vi "飞行姿态模拟.vi"() -> ()   [LabVIEW 2014]
uses:
  <vilib>/Utility/miscctls.llb/LVRGBAColorTypeDef.ctl
  <vilib>/picture/3D Picture Control/Object/Create Object (name).vi
  <vilib>/picture/3D Picture Control/Object/Add Object (reference).vi
  <vilib>/picture/3D Picture Control/NI_3D Picture Control.lvlib
panel:
  in  "退出按钮":bool
  in  "Yaw":dbl(knob) scale=-180.0..180.0
  in  "Roll":dbl(knob) scale=-90.0..90.0
  in  "Pitch":dbl(knob) scale=-180.0..180.0
  out "三维图片":refnum<vi>(3d-picture)
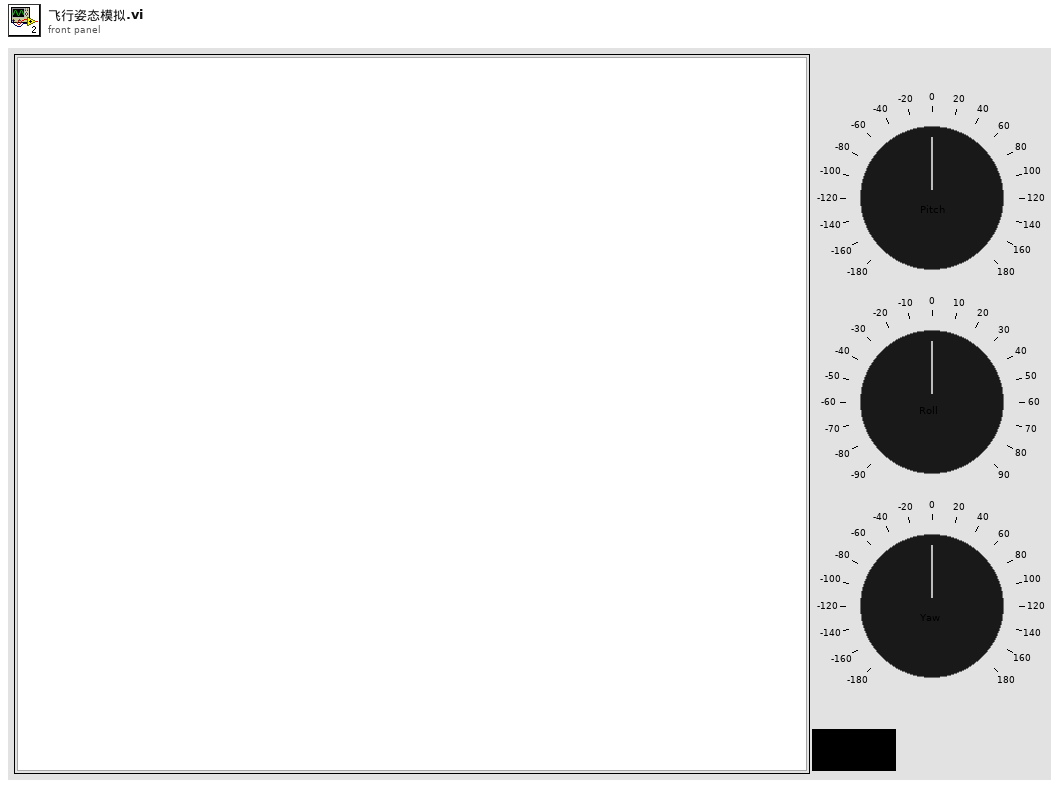
[diagram p1: front panel]
types:
  T1 = typedef "LVRGBAColorTypeDef.ctl" = cluster{"Red":sgl, "Green":sgl, "Blue":sgl, "Alpha":sgl}
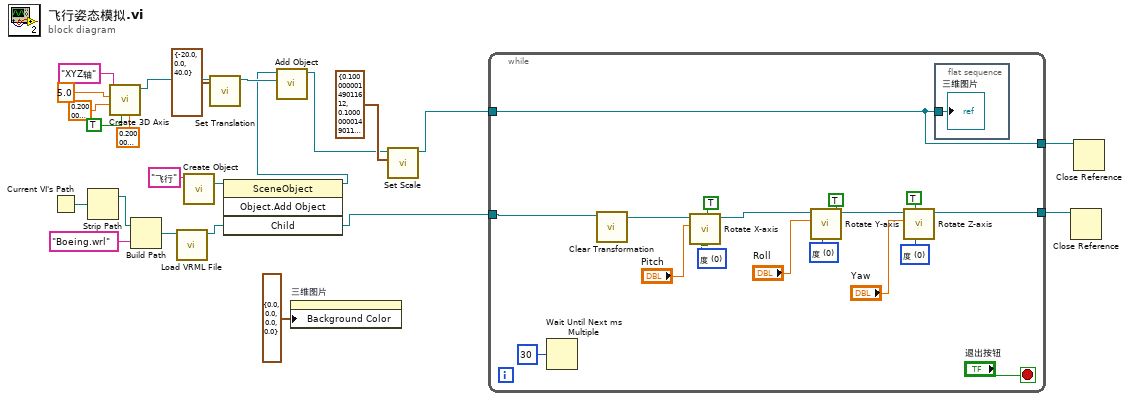
[diagram p0: block diagram]
diagram:
  n1 = Current VI's Path() -> (path=w21:path)
  n2 = Strip Path ("拆分路径")(path=w21) -> (stripped path=w20:path)  [unwired: 1 out]
  n3 = call <vilib>:"Create 3D Axis.vi"("Character Size"=sgl 0.2, "Axis label?"=TRUE, "Radius"=sgl 0.2, "Length"=sgl 5.0, "Name"="XYZ轴") -> ("New Object Refnum"=w6:refnum<vi>)  [unwired: 5 in, 1 out]
  n4 = Build Path ("创建路径")(base path=w20, name or relative path="Boeing.wrl" ("名称或相对路径")) -> (appended path=w18:path)
  n5 = call <vilib>:"Load VRML File.vi"("Path"=w18) -> ("Scene:Read Scene File"=w14:refnum<vi>)  [unwired: 9 in, 1 out]
  n6 = call-poly <vilib>:"Create Object.vi"("Name"="飞行") -> ("Scene:New Object"=w17:refnum<vi>)  [unwired: 9 in, 1 out]
  n7 = call <vilib>:"Set Translation.vi"("Translation"=cluster{"X":sgl, "Y":sgl, "Z":sgl} {"X"=-20.0, "Y"=0.0, "Z"=40.0}, "Scene Object"=w6) -> ("Translated Object"=w5:refnum<vi>)  [unwired: 8 in, 1 out]
  n8 = invoke class="SceneObject" method="Object.Add Object"(reference=w17, "Child"=w14) -> (reference out=w4:refnum<vi>, "Child"=w3:refnum<vi>)  [unwired: 2 in, 2 out]
  n9 = call-poly <vilib>:"Add Object.vi"("New Object In"=w5, "Scene Object In"=w4) -> ("Scene Object Out"=w7:refnum<vi>)  [unwired: 7 in, 2 out]
  n10 = property on="三维图片" class="SceneGraphDisp (严格)"("Background Color"=T1 {"Red"=0.0, "Green"=0.0, "Blue"=0.0, "Alpha"=0.0} ("背景色")) -> ()  [unwired: 2 in, 2 out]
  n11 = call <vilib>:"Set Scale.vi"("Scale"=cluster{"X":sgl, "Y":sgl, "Z":sgl} {"X"=0.1, "Y"=0.1, "Z"=0.1}, "Scene Object"=w7) -> ("Scaled Object"=w2:refnum<vi>)  [unwired: 8 in, 1 out]
  n12 = while {
    tunnel: w2 -> [w31]
    tunnel: w3 -> [w32]
    tunnel: [w31] -> w23
    tunnel: [w30] -> w22
    stop <- "退出按钮" stop-if-true
    w37 = u16 0 items=["度", "弧度"] ("angle unit")
    w38 = u16 0 items=["度", "弧度"] ("angle unit")
    w39 = u16 0 items=["度", "弧度"] ("angle unit")
    n13 = Wait Until Next ms Multiple(millisecond multiple=u32 30 ("毫秒倍数")) -> ()  [unwired: 1 out]
    n14 = call <vilib>:"Clear Transformation.vi"("Object Refnum In"=w32) -> ("Object Refnum Out"=w34:refnum<vi>)  [unwired: 9 in, 1 out]
    n15 = call <vilib>:"Rotate X-axis.vi"("angle unit"=w39, "Relative?"=TRUE, "angle"="Pitch", "Scene Object In"=w34) -> ("Scene Object Out"=w36:refnum<vi>)  [unwired: 6 in, 1 out]
    n16 = call <vilib>:"Rotate Y-axis.vi"("angle unit"=w38, "Relative?"=TRUE, "angle"="Roll", "Scene Object In"=w36) -> ("Scene Object Out"=w35:refnum<vi>)  [unwired: 6 in, 1 out]
    n17 = call <vilib>:"Rotate Z-axis.vi"("angle unit"=w37, "Relative?"=TRUE, "angle"="Yaw", "Scene Object In"=w35) -> ("Scene Object Out"=w30:refnum<vi>)  [unwired: 6 in, 1 out]
    n18 = flat-sequence {
      tunnel: w31 -> [w41]
      frame #0 {
        "三维图片" <- w41
      }
    }
  }
  n19 = Close Reference(reference=w22) -> ()  [unwired: 1 in, 1 out]
  n20 = Close Reference(reference=w23) -> ()  [unwired: 1 in, 1 out]
